vi "String to Lat Lon (SubVI).vi"(2 "EW":string, 3 "Longitude":string, 4 "N S":string, 5 "Latitude":string) -> (0 "Lon":string, 1 "Lat":string)   [LabVIEW 2012]
uses:
  <vilib>/regexp/Match Regular Expression.xnode
panel:
  out "before match":string
  out "Numeric 2":i32
  out "mm":dbl
  out "mm":string
  out "degrees":i32
  out "degrees":string
  out "Numeric":i32
  out "mm":dbl
  out "mm":string
  out "degrees":i32
  out "degrees":string
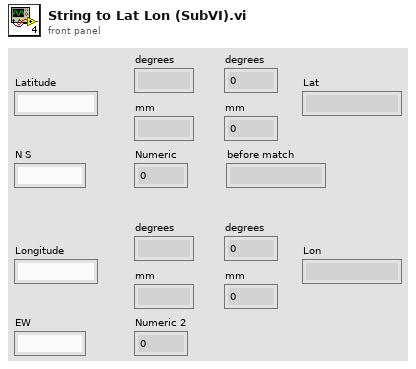
[diagram p1: front panel]
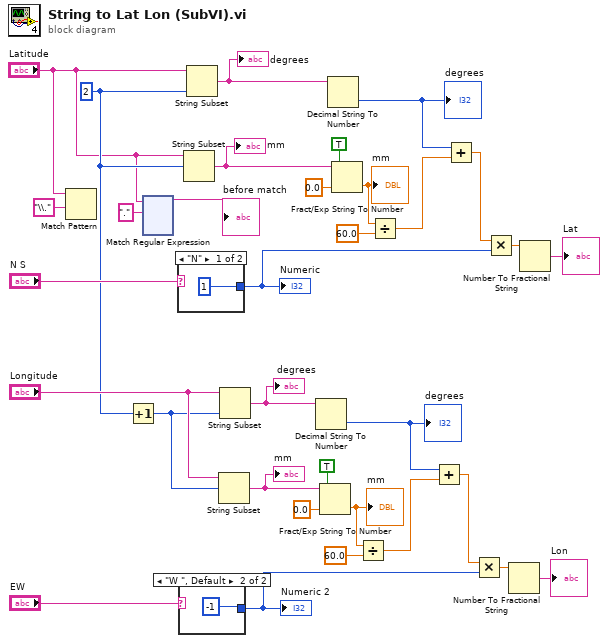
[diagram p0: block diagram]
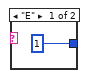
[diagram p2: hidden frame]
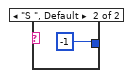
[diagram p3: hidden frame]
diagram:
  w10 = 2 ("length (rest)")
  n1 = Match Pattern(string="Latitude", regular expression="\\.") -> ()  [unwired: 1 in, 4 out]
  n2 = Increment(x=w10) -> (x+1=w9:i32)
  n3 = xnode "Match Regular Expression"("input string"="Latitude", "regular expression"=".") -> ("before match"=→"before match":string)  [unwired: 4 in, 4 out]
  n4 = case shown="\"N\"" "N S" {
    tunnel: [1 -1] -> w25
    frame "N" {
    }
    frame "S ", Default {
    }
  }
  "Numeric" <- w25
  n5 = case shown="\"W \", Default" "EW" {
    tunnel: [1 -1] -> w14
    frame "E" {
    }
    frame "W ", Default {
    }
  }
  "Numeric 2" <- w14
  n6 = String Subset(string="Latitude", offset (0)=w10) -> (substring=w31:string)  [unwired: 1 in]
  "mm" <- w31
  n7 = String Subset(string="Latitude", length (rest)=w10) -> (substring=w33:string)  [unwired: 1 in]
  "degrees" <- w33
  n8 = String Subset(string="Longitude", offset (0)=w9) -> (substring=w20:string)  [unwired: 1 in]
  "mm" <- w20
  n9 = String Subset(string="Longitude", length (rest)=w9) -> (substring=w23:string)  [unwired: 1 in]
  "degrees" <- w23
  n10 = Decimal String To Number(string=w23) -> (number=w12:i32)  [unwired: 2 in, 1 out]
  "degrees" <- w12
  n11 = Fract/Exp String To Number(use system decimal point (T)=TRUE, string=w20, default (0 dbl)=0.0 ("default (0 DBL)")) -> (number=w17:dbl)  [unwired: 1 in, 1 out]
  "mm" <- w17
  n12 = Decimal String To Number(string=w33) -> (number=w11:i32)  [unwired: 2 in, 1 out]
  "degrees" <- w11
  n13 = Fract/Exp String To Number(use system decimal point (T)=TRUE, string=w31, default (0 dbl)=0.0 ("default (0 DBL)")) -> (number=w28:dbl)  [unwired: 1 in, 1 out]
  "mm" <- w28
  n14 = Divide(x=w17, y=60.0) -> (x/y=w15:dbl)
  n15 = Divide(x=w28, y=60.0) -> (x/y=w26:dbl)
  n16 = Add(x=w12, y=w15) -> (x+y=w13:dbl)
  n17 = Add(x=w11, y=w26) -> (x+y=w24:dbl)
  n18 = Multiply(x=w13, y=w14) -> (x*y=w5:dbl)
  n19 = Multiply(x=w24, y=w25) -> (x*y=w7:dbl)
  n20 = Number To Fractional String(number=w5) -> (F-format string=→"Lon":string)  [unwired: 3 in]
  n21 = Number To Fractional String(number=w7) -> (F-format string=→"Lat":string)  [unwired: 3 in]
